vi "Timing.Set Iteration.vi"(10 "Iteration":u64=1, 11 "Timing in":refnum<class "Timing.lvclass">) -> (3 "Timing out":refnum<class "Timing.lvclass">)   [LabVIEW 2017, in "DSF.Engine.lvlib" / "Timing.lvclass"]
uses:
  Timing.lvclass
  Timing.lvclass/Timing.ctl
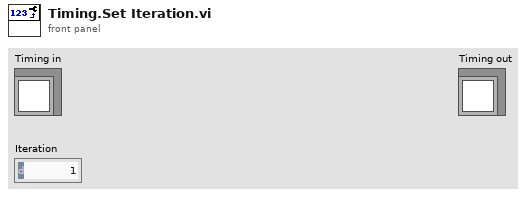
[diagram p1: front panel]
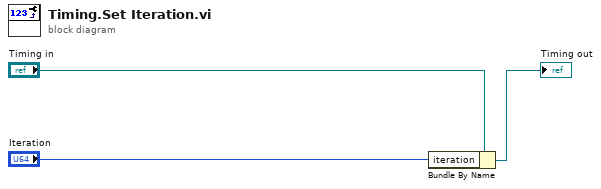
[diagram p0: block diagram]
diagram:
  n1 = Bundle By Name(cluster="Timing in", "iteration"="Iteration") -> (→"Timing out":refnum<class "Timing.lvclass">)
